vi "calcEncoderPosition.vi"(8 "error in (no error)":errorcluster, 11 "EnccoderConverter in":refnum<class "EncoderConverter.lvclass">) -> (0 "error out":errorcluster, 3 "EnccoderConverter out":refnum<class "EncoderConverter.lvclass">)   [LabVIEW 2013, in "EncoderConverter.lvlib" / "EncoderConverter.lvclass"]
uses:
  <userlib>/Common/Devices/EncoderConverter/EncoderConverter/EncoderConverter.lvclass
  <userlib>/Common/Devices/EncoderConverter/EncoderConverter/EncoderConverter.lvclass/EncoderConverter.ctl
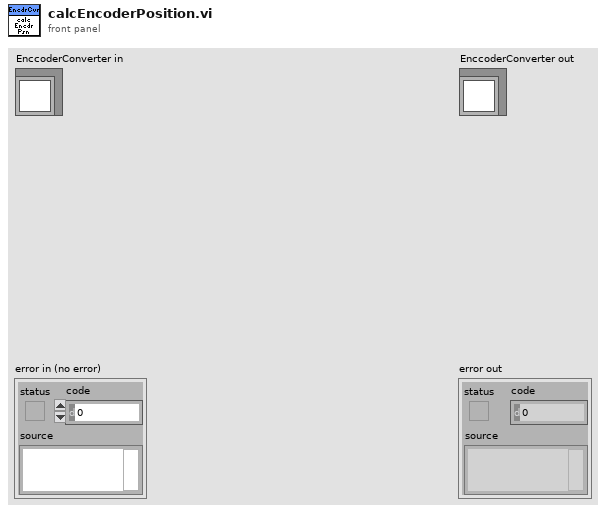
[diagram p1: front panel]
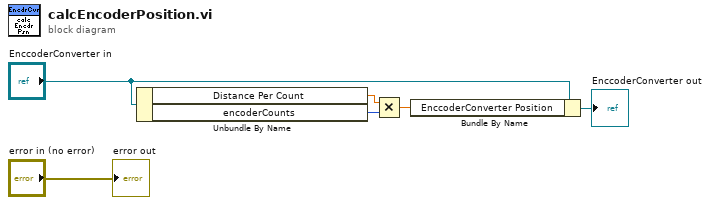
[diagram p0: block diagram]
diagram:
  n1 = Unbundle By Name("EnccoderConverter in") -> ("Distance Per Count"=w5:dbl[unit], "encoderCounts"=w4:i32)
  n2 = Multiply(x=w5, y=w4) -> (x*y=w1:dbl[unit])
  n3 = Bundle By Name(cluster="EnccoderConverter in", "EnccoderConverter Position"=w1) -> (→"EnccoderConverter out":refnum<class "EncoderConverter.lvclass">)
  "error out" <- "error in (no error)"
